vi "removeU-Inois.vi"(5 "I-nois subtr.":bool, 7 "U-nois subtr.":bool, 10 "Array in":waveform(dbl)[](array[waveform]), 11 "data info template":refnum<vi>) -> (3 "Array out":waveform(dbl)[](array[waveform]))   [LabVIEW 2014]
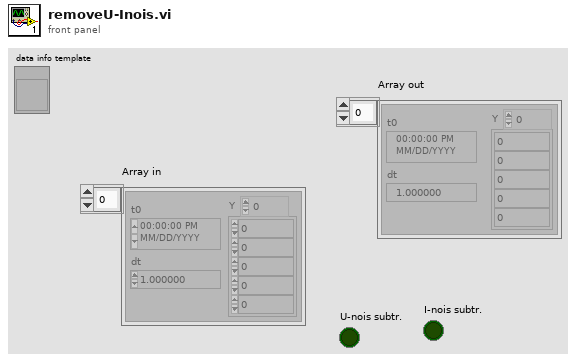
[diagram p1: front panel]
types:
  T1 = cluster{"data path":string, "ADCintercadr_s":dbl, "data info":cluster{"use or not *.info.txt?":i16, "probe name":string, "signal type":string, "Unit":string, "variable":string, "attenuation factor":dbl, "amplification factor":dbl, "extracoef#1":dbl, "extracoef#2":dbl, "U cascade, kV":string, "probe area, cm2":dbl, "plasma, a.m.u.":dbl}, "channel_name":string, "channels_in_file":i32}
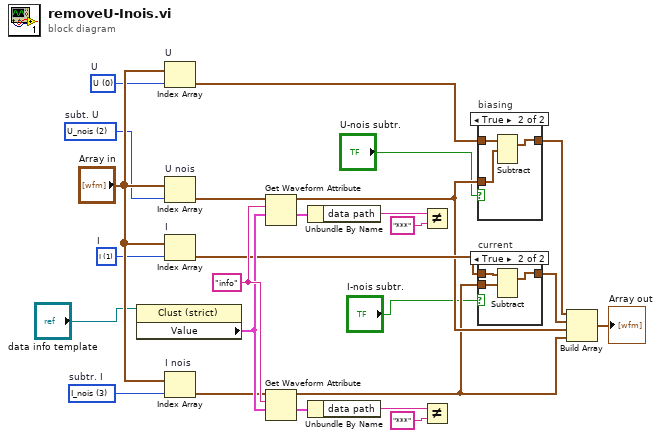
[diagram p0: block diagram]
diagram:
  w21 = "info" ("name")
  w9 = u16 1 items=["U", "I", "U_nois", "I_nois"]  # I
  w8 = u16 0 items=["U", "I", "U_nois", "I_nois"]  # U
  w7 = u16 3 items=["U", "I", "U_nois", "I_nois", ""]  # subtr. I
  w6 = u16 2 items=["U", "I", "U_nois", "I_nois"]  # subt. U
  n1 = property class="Clust (strict)"(reference="data info template") -> ("Value"=w16:T1)  [unwired: 1 in, 2 out]
  n2 = Index Array "U"(array="Array in", index=w8) -> (element=w10:waveform(dbl))
  n3 = Index Array "U nois"(array="Array in", index=w6) -> (element=w12:waveform(dbl))
  n4 = Index Array "I"(array="Array in", index=w9) -> (element=w11:waveform(dbl))
  n5 = Index Array "I nois"(array="Array in", index=w7) -> (element=w15:waveform(dbl))
  n6 = Get Waveform Attribute(5:w16, 6:w21, 7:w12) -> (1:w13:T1, 3:w5:waveform(dbl))  [unwired: 1 in, 2 out]
  n7 = Get Waveform Attribute(5:w16, 6:w21, 7:w15) -> (1:w14:T1, 3:w4:waveform(dbl))  [unwired: 1 in, 2 out]
  n8 = Unbundle By Name(w13) -> ("data path"=w17:string)
  n9 = Unbundle By Name(w14) -> ("data path"=w20:string)
  n10 = Not Equal?(x=w17, y="***") -> ()  [unwired: 1 out]
  n11 = Not Equal?(x=w20, y="***") -> ()  [unwired: 1 out]
  n12 = case "biasing" shown="True" "U-nois subtr." {
    tunnel: w10 -> [w26 w29]
    tunnel: w5 -> [_ w28]
    tunnel: [w26 w27] -> w23
    frame False {
    }
    frame True {
      n13 = Subtract(1:w28, 2:w29) -> (0:w27:waveform(dbl))  [unwired: 1 in, 1 out]
    }
  }
  n14 = case "current" shown="True" "I-nois subtr." {
    tunnel: w11 -> [w30 w33]
    tunnel: w4 -> [_ w32]
    tunnel: [w30 w31] -> w24
    frame False {
    }
    frame True {
      n15 = Subtract(1:w32, 2:w33) -> (0:w31:waveform(dbl))  [unwired: 1 in, 1 out]
    }
  }
  n16 = Build Array(w23, w24, w5, w4) -> (→"Array out":waveform(dbl)[])
